vi "JoystickFunctionL (SubVI).vi"(6 "TimeToReachSpeed":dbl, 7 "DeltaT":dbl, 9 "TweenedSpeed":dbl, 10 "DesiredSpeed":dbl) -> (3 "OutputMotorValueL":dbl)   [LabVIEW 2012]
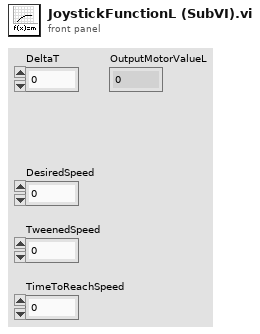
[diagram p1: front panel]
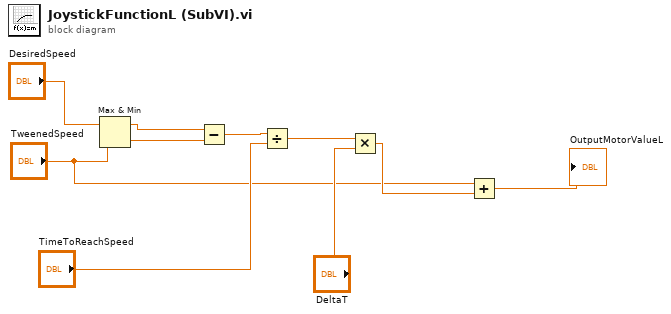
[diagram p0: block diagram]
diagram:
  n1 = Max & Min(x="DesiredSpeed", y="TweenedSpeed") -> (max(x,y)=w3:dbl, min(x,y)=w4:dbl)
  n2 = Subtract(x=w3, y=w4) -> (x-y=w5:dbl)
  n3 = Divide(x=w5, y="TimeToReachSpeed") -> (x/y=w6:dbl)
  n4 = Multiply(x=w6, y="DeltaT") -> (x*y=w9:dbl)
  n5 = Add(x="TweenedSpeed", y=w9) -> (x+y=→"OutputMotorValueL":dbl)
